vi "Ejercicio 3.1.vi"() -> ()   [LabVIEW 2021]
panel:
  out "Array":dbl[](array[numeric])
  in  "N1":dbl
  in  "N2":dbl
  out "A":dbl[](array[numeric])
  out "B":dbl[](array[numeric])
  in  "X":dbl
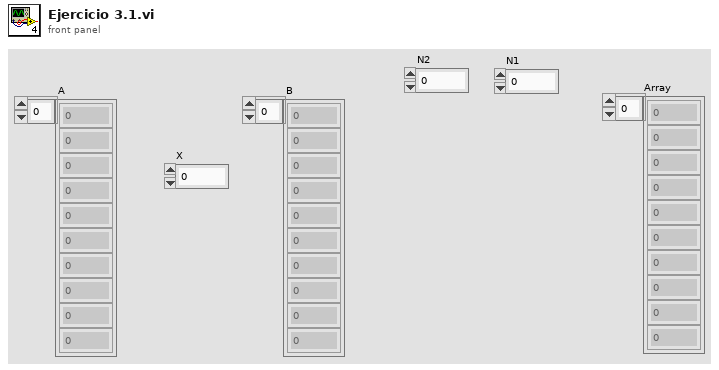
[diagram p1: front panel]
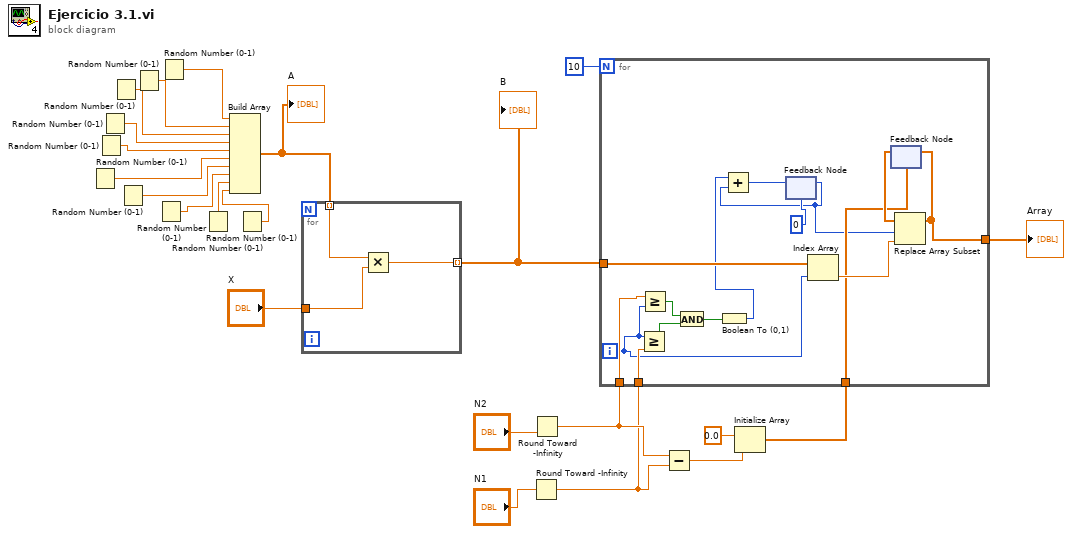
[diagram p0: block diagram]
diagram:
  n1 = Random Number (0-1)() -> (number: 0 to 1=w17:dbl)
  n2 = Random Number (0-1)() -> (number: 0 to 1=w18:dbl)
  n3 = Random Number (0-1)() -> (number: 0 to 1=w19:dbl)
  n4 = Random Number (0-1)() -> (number: 0 to 1=w20:dbl)
  n5 = Random Number (0-1)() -> (number: 0 to 1=w16:dbl)
  n6 = Random Number (0-1)() -> (number: 0 to 1=w21:dbl)
  n7 = Random Number (0-1)() -> (number: 0 to 1=w15:dbl)
  n8 = Random Number (0-1)() -> (number: 0 to 1=w22:dbl)
  n9 = Random Number (0-1)() -> (number: 0 to 1=w14:dbl)
  n10 = Random Number (0-1)() -> (number: 0 to 1=w13:dbl)
  n11 = Build Array(w22, w21, w20, w19, w18, w17, w16, w15, w14, w13) -> (w11:dbl[])
  "A" <- w11
  n12 = for {
    tunnel: w11 -> [w25] mode=indexing
    tunnel: "X" -> [w24]
    tunnel: [w23] -> w6 mode=indexing
    n13 = Multiply(x=w25, y=w24) -> (x*y=w23:dbl)
  }
  "B" <- w6
  n14 = Round Toward -Infinity(1:"N1") -> (0:w7:dbl)
  n15 = Round Toward -Infinity(1:"N2") -> (0:w8:dbl)
  n16 = Subtract(x=w8, y=w7) -> (x-y=w2:dbl)
  n17 = Initialize Array(0.0, w2) -> (w3:dbl[])
  n18 = for {
    N: 10 -> [_]
    tunnel: w8 -> [w30]
    tunnel: w7 -> [w29]
    tunnel: w6 -> [w37]
    tunnel: w3 -> [w33]
    tunnel: [w32] -> w1
    i -> [w28]
    n19 = Greater Or Equal?(x=w28, y=w29) -> (x >= y?=w26:bool)
    n20 = Greater Or Equal?(x=w30, y=w28) -> (x >= y?=w27:bool)
    n21 = And(x=w27, y=w26) -> (x .and. y?=w39:bool)
    n22 = Boolean To (0,1)(Boolean=w39) -> (0, 1=w34:i16)
    n23 = feedback #1(0) -> (w31:i32)
    n24 = Add(x=w34, y=w31) -> (x+y=w35:i32)
    n25 = feedback-in #1(w35) -> ()
    n26 = Index Array(array=w37, index=w28) -> (element=w36:dbl)
    n27 = feedback #2(w33) -> (w38:dbl[])
    n28 = Replace Array Subset(array=w38, new element=w36, index=w31) -> (w32:dbl[])
    n29 = feedback-in #2(w32) -> ()
  }
  "Array" <- w1
